vi "highpass_image_Widefield_hacked.vi"(8 "Spatial filter size (um)":i32=5, 11 "Image":T1) -> (3 "high passed image":T1)   [LabVIEW 2014]
uses:
  <vilib>/vision/Image Controls.llb/IMAQ Image.ctl
  Widefield_globals.vi
  <vilib>/gmath/interp.llb/Interpolate 2D (1d xi,yi).vi
  <vilib>/vision/NI_Vision_Development_Module.lvlib
  <vilib>/gmath/NI_Gmath.lvlib
panel:
  in  "Gauss size":i32=45
  in  "gauss21":sgl[][](array[numeric])=[[0.000334, 0.000433, 0.000547, 0.000672, 0.000803, 0.000934, 0.001056, 0.001162, 0.001245, 0.001297, 0.001315, 0.001297, 0.001245, 0.001162, 0.001056, 0.000934, 0.000803, 0.000672, 0.000547, 0.000433, 0.000334], [0.000433, 0.000562, 0.00071, 0.000872, 0.001042, 0.001211, 0.00137, 0.001508, 0.001615, 0.001682, 0.001705, 0.001682, 0.001615, 0.001508, 0.00137, 0.001211, 0.001042, 0.000872, 0.00071, 0.000562, 0.000433], [0.000547, 0.00071, 0.000896, 0.0011, 0.001315, 0.001528, 0.001729, 0.001903, 0.002038, 0.002123, 0.002152, 0.002123, 0.002038, 0.001903, 0.001729, 0.001528, 0.001315, 0.0011, 0.000896, 0.00071, 0.000547], [0.000672, 0.000872, 0.0011, 0.001351, 0.001615, 0.001877, 0.002123, 0.002337, 0.002502, 0.002607, 0.002643, 0.002607, 0.002502, 0.002337, 0.002123, 0.001877, 0.001615, 0.001351, 0.0011, 0.000872, 0.000672], [0.000803, 0.001042, 0.001315, 0.001615, 0.001929, 0.002243, 0.002537, 0.002792, 0.00299, 0.003115, 0.003158, 0.003115, 0.00299, 0.002792, 0.002537, 0.002243, 0.001929, 0.001615, 0.001315, 0.001042, 0.000803], [0.000934, 0.001211, 0.001528, 0.001877, 0.002243, 0.002607, 0.002949, 0.003246, 0.003476, 0.003621, 0.003671, 0.003621, 0.003476, 0.003246, 0.002949, 0.002607, 0.002243, 0.001877, 0.001528, 0.001211, 0.000934], [0.001056, 0.00137, 0.001729, 0.002123, 0.002537, 0.002949, 0.003336, 0.003671, 0.003931, 0.004096, 0.004153, 0.004096, 0.003931, 0.003671, 0.003336, 0.002949, 0.002537, 0.002123, 0.001729, 0.00137, 0.001056], [0.001162, 0.001508, 0.001903, 0.002337, 0.002792, 0.003246, 0.003671, 0.004041, 0.004327, 0.004508, 0.00457, 0.004508, 0.004327, 0.004041, 0.003671, 0.003246, 0.002792, 0.002337, 0.001903, 0.001508, 0.001162], [0.001245, 0.001615, 0.002038, 0.002502, 0.00299, 0.003476, 0.003931, 0.004327, 0.004633, 0.004828, 0.004894, 0.004828, 0.004633, 0.004327, 0.003931, 0.003476, 0.00299, 0.002502, 0.002038, 0.001615, 0.001245], [0.001297, 0.001682, 0.002123, 0.002607, 0.003115, 0.003621, 0.004096, 0.004508, 0.004828, 0.00503, 0.005099, 0.00503, 0.004828, 0.004508, 0.004096, 0.003621, 0.003115, 0.002607, 0.002123, 0.001682, 0.001297], [0.001315, 0.001705, 0.002152, 0.002643, 0.003158, 0.003671, 0.004153, 0.00457, 0.004894, 0.005099, 0.00517, 0.005099, 0.004894, 0.00457, 0.004153, 0.003671, 0.003158, 0.002643, 0.002152, 0.001705, 0.001315], [0.001297, 0.001682, 0.002123, 0.002607, 0.003115, 0.003621, 0.004096, 0.004508, 0.004828, 0.00503, 0.005099, 0.00503, 0.004828, 0.004508, 0.004096, 0.003621, 0.003115, 0.002607, 0.002123, 0.001682, 0.001297], [0.001245, 0.001615, 0.002038, 0.002502, 0.00299, 0.003476, 0.003931, 0.004327, 0.004633, 0.004828, 0.004894, 0.004828, 0.004633, 0.004327, 0.003931, 0.003476, 0.00299, 0.002502, 0.002038, 0.001615, 0.001245], [0.001162, 0.001508, 0.001903, 0.002337, 0.002792, 0.003246, 0.003671, 0.004041, 0.004327, 0.004508, 0.00457, 0.004508, 0.004327, 0.004041, 0.003671, 0.003246, 0.002792, 0.002337, 0.001903, 0.001508, 0.001162], [0.001056, 0.00137, 0.001729, 0.002123, 0.002537, 0.002949, 0.003336, 0.003671, 0.003931, 0.004096, 0.004153, 0.004096, 0.003931, 0.003671, 0.003336, 0.002949, 0.002537, 0.002123, 0.001729, 0.00137, 0.001056], [0.000934, 0.001211, 0.001528, 0.001877, 0.002243, 0.002607, 0.002949, 0.003246, 0.003476, 0.003621, 0.003671, 0.003621, 0.003476, 0.003246, 0.002949, 0.002607, 0.002243, 0.001877, 0.001528, 0.001211, 0.000934], [0.000803, 0.001042, 0.001315, 0.001615, 0.001929, 0.002243, 0.002537, 0.002792, 0.00299, 0.003115, 0.003158, 0.003115, 0.00299, 0.002792, 0.002537, 0.002243, 0.001929, 0.001615, 0.001315, 0.001042, 0.000803], [0.000672, 0.000872, 0.0011, 0.001351, 0.001615, 0.001877, 0.002123, 0.002337, 0.002502, 0.002607, 0.002643, 0.002607, 0.002502, 0.002337, 0.002123, 0.001877, 0.001615, 0.001351, 0.0011, 0.000872, 0.000672], [0.000547, 0.00071, 0.000896, 0.0011, 0.001315, 0.001528, 0.001729, 0.001903, 0.002038, 0.002123, 0.002152, 0.002123, 0.002038, 0.001903, 0.001729, 0.001528, 0.001315, 0.0011, 0.000896, 0.00071, 0.000547], [0.000433, 0.000562, 0.00071, 0.000872, 0.001042, 0.001211, 0.00137, 0.001508, 0.001615, 0.001682, 0.001705, 0.001682, 0.001615, 0.001508, 0.00137, 0.001211, 0.001042, 0.000872, 0.00071, 0.000562, 0.000433], [0.000334, 0.000433, 0.000547, 0.000672, 0.000803, 0.000934, 0.001056, 0.001162, 0.001245, 0.001297, 0.001315, 0.001297, 0.001245, 0.001162, 0.001056, 0.000934, 0.000803, 0.000672, 0.000547, 0.000433, 0.000334]] format="%0.3f"
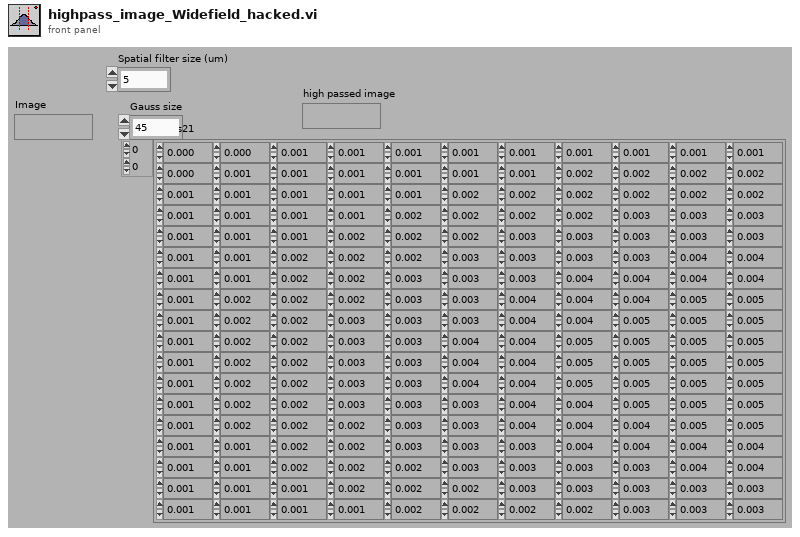
[diagram p1: front panel]
types:
  T1 = typedef "IMAQ Image.ctl" = refnum<image>
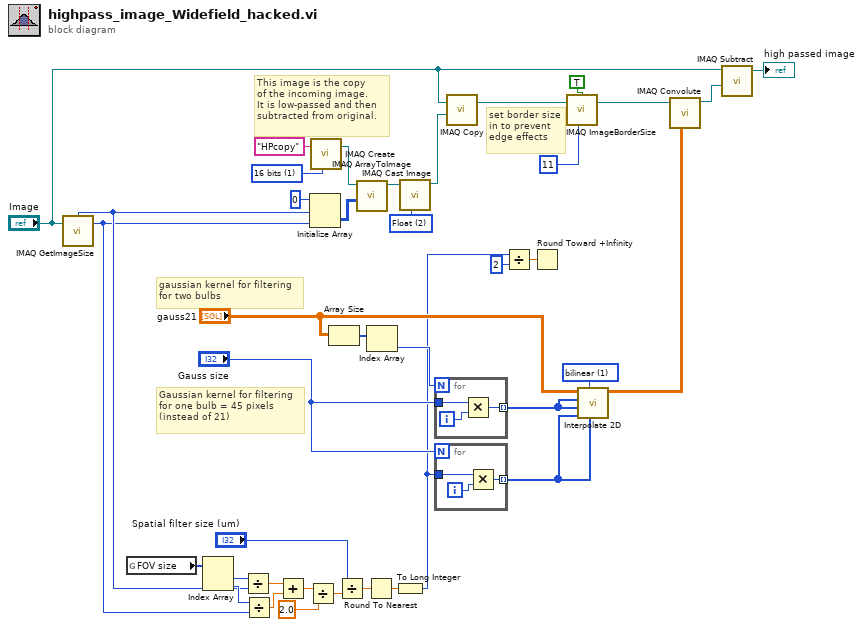
[diagram p0: block diagram]
diagram:
  w26 = 1 items=["nearest", "bilinear", "bicubic", "bicubic spline"] ("method")
  w23 = u32 2 items=["8 bits", "16 bits", "Float", "Complex", "RGB", "HSL"] ("Image Type")
  w37 = u32 1 items=["8 bits", "16 bits", "Float", "Complex", "RGB", "HSL"] ("Image Type")
  # "gaussian kernel for filtering\nfor two bulbs"
  # "Gaussian kernel for filtering\nfor one bulb = 45 pixels\n(instead of 21)"
  # "set border size\nin to prevent\nedge effects"
  # "This image is the copy \nof the incoming image. \nIt is low-passed and then\nsubtracted from original."
  n1 = call "IMAQ GetImageSize"("Image"="Image") -> ("Y Resolution"=w4:i32, "X Resolution"=w5:i32)  [unwired: 1 in, 3 out]
  n2 = global read "Widefield_globals.vi" "FOV size"() -> (w16:i32[])
  n3 = Index Array(array=w16) -> (element #1=w15:i32, element #2=w14:i32)  [unwired: 2 in]
  n4 = Divide(x=w15, y=w5) -> (x/y=w13:dbl)
  n5 = Divide(x=w14, y=w4) -> (x/y=w12:dbl)
  n6 = Add(x=w13, y=w12) -> (x+y=w11:dbl)
  n7 = Divide(x=w11, y=2.0) -> (x/y=w9:dbl)
  n8 = Initialize Array(0, w5, w4) -> (w36:i32[][])
  n9 = call "IMAQ Create"("Image Name"="HPcopy", "Image Type"=w37) -> ("New Image"=w38:T1)  [unwired: 2 in, 2 out]
  n10 = Array Size(array="gauss21") -> (size(s)=w18:i32[])
  n11 = Divide(x="Spatial filter size (um)", y=w9) -> (x/y=w7:dbl)
  n12 = call "IMAQ ArrayToImage"("Image Pixels (I16)"=w36, "Image"=w38) -> ("Image Out"=w35:T1)  [unwired: 4 in, 5 out]
  n13 = Round To Nearest(number=w7) -> (nearest integer value=w6:dbl)
  n14 = Index Array(array=w18) -> (element=w17:i32)  [unwired: 1 in]
  n15 = To Long Integer(number=w6) -> (32bit integer=w2:i32)
  n16 = call "IMAQ Cast Image"("Image Type"=w23, "Image Src"=w35) -> ("Image Dst Out"=w33:T1)  [unwired: 4 in, 5 out]
  n17 = for {
    N: w17 -> [_]
    tunnel: [w41] -> w25 mode=indexing
    tunnel: "Gauss size" -> [w40]
    i -> [w42]
    n18 = Multiply(x=w40, y=w42) -> (x*y=w41:i32)
  }
  n19 = for {
    N: "Gauss size" -> [_]
    tunnel: [w44] -> w24 mode=indexing
    tunnel: w2 -> [w43]
    i -> [w45]
    n20 = Multiply(x=w43, y=w45) -> (x*y=w44:i32)
  }
  n21 = call "IMAQ Copy"("Image Dst"=w33, "Image Src"="Image") -> ("Image Dst Out"=w29:T1)  [unwired: 1 in, 4 out]
  n22 = Divide(x=w2, y=2) -> (x/y=w21:dbl)
  n23 = Round Toward +Infinity(x=w21) -> ()  [unwired: 1 out]
  n24 = call "IMAQ ImageBorderSize"("Get/Set Status? (Set)"=TRUE, "Image"=w29, "Image border size in"=11) -> ("Image Out"=w28:T1)  [unwired: 1 in, 2 out]
  n25 = call-poly <vilib>:"Interpolate 2D.vi"("yi"=w24, "method"=w26, "xi"=w24, "Y"=w25, "X"=w25, "Z"="gauss21") -> ("zi"=w3:dbl[][])  [unwired: 1 in, 4 out]
  n26 = call "IMAQ Convolute"("Kernel"=w3, "Image Src"=w28) -> ("Image Dst Out"=w31:T1)  [unwired: 5 in, 4 out]
  n27 = call "IMAQ Subtract"("Image Src A"="Image", "Image Src B"=w31) -> ("Image Dst Out"=→"high passed image":T1)  [unwired: 3 in, 3 out]
